vi "23384_Davis_Poku_Amankwa_Amankwa.DavisPoku.MNE1201.8.DIY_348265_461660684.vi"() -> ()   [LabVIEW 2018]
panel:
  out "Reaction Time(ms)":dbl
  out "Square Led":bool
  in  "?":bool
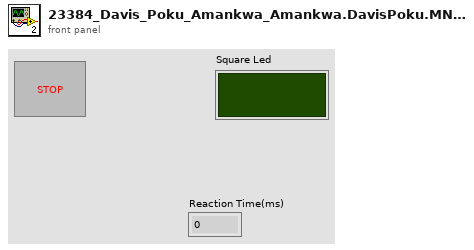
[diagram p1: front panel]
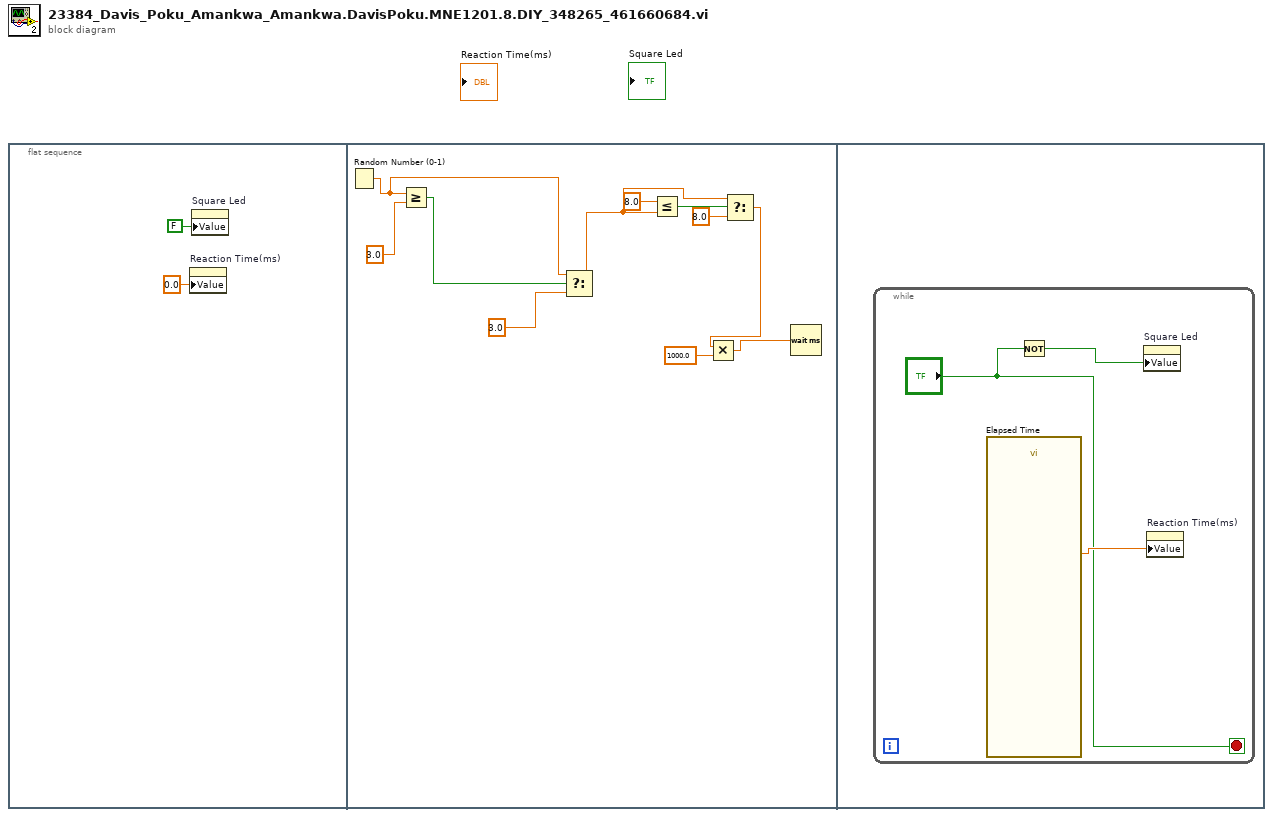
[diagram p0: block diagram]
diagram:
  n1 = flat-sequence {
    frame #0 {
      n2 = property on="Reaction Time(ms)" class="DigNum (strict)"("Value"=0.0 ("Reaction Time(ms)")) -> ()  [unwired: 2 in, 2 out]
      n3 = property on="Square Led" class="Bool (strict)"("Value"=FALSE ("Square Led")) -> ()  [unwired: 2 in, 2 out]
    }
    frame #1 {
      n4 = Random Number (0-1)() -> (number: 0 to 1=w9:dbl)
      n5 = Greater Or Equal?(x=w9, y=3.0) -> (x >= y?=w12:bool)
      n6 = Select(t=w9, s=w12, f=3.0) -> (s? t:f=w6:dbl)
      n7 = Less Or Equal?(x=8.0, y=w6) -> (x <= y?=w7:bool)
      n8 = Select(t=w6, s=w7, f=8.0) -> (s? t:f=w4:dbl)
      n9 = Multiply(x=w4, y=1000.0) -> (x*y=w3:dbl)
      n10 = Wait (ms)(milliseconds to wait=w3) -> ()  [unwired: 1 out]
    }
    frame #2 {
      n11 = while {
        stop <- "?" stop-if-true
        n12 = call "Elapsed Time"() -> ("Elapsed Time (s)"=w16:dbl)  [unwired: 12 in, 7 out]
        n13 = Not(x="?") -> (.not. x?=w14:bool)
        n14 = property on="Square Led" class="Bool (strict)"("Value"=w14) -> ()  [unwired: 2 in, 2 out]
        n15 = property on="Reaction Time(ms)" class="DigNum (strict)"("Value"=w16) -> ()  [unwired: 2 in, 2 out]
      }
    }
  }
